vi "Setup measurement.vi"(7 "PLC (2)":dbl=2.0 format="%#_13g", 8 "error in (no error)":errorcluster, 10 "Source Limit Level (0.1)":dbl=0.1, 11 "VISA Refnum in":refnum<visa-resource-name>) -> (0 "error in (no error) 2":errorcluster, 3 "VISA resource name out":refnum<visa-resource-name>)   [LabVIEW 2021]
uses:
  <instrlib>/Keithley 2450/Keithley 2450.lvlib
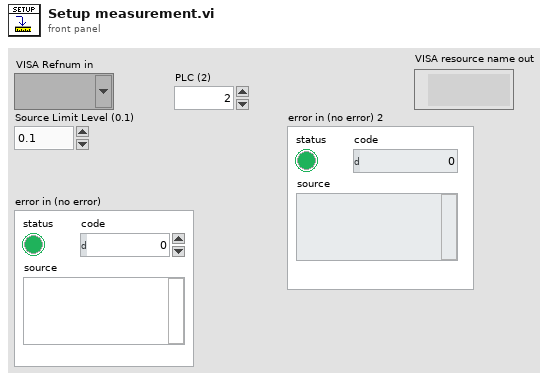
[diagram p1: front panel]
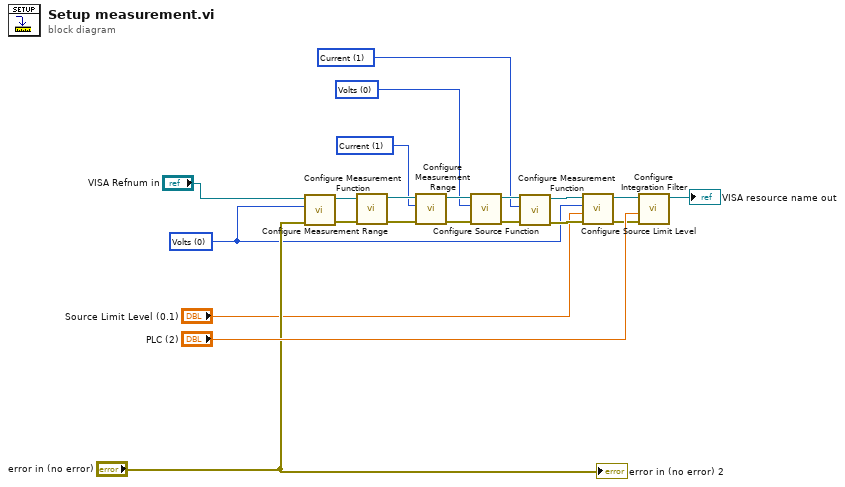
[diagram p0: block diagram]
diagram:
  w3 = u16 1 items=["Volts", "Current", "Resistance"] ("Function (0: Volts)")
  w5 = u16 0 items=["Volts", "Current"] ("Function (0: Volts)")
  w6 = u16 1 items=["Volts", "Current", "Auto Resistance", "Manual Resistance", "Digitize Voltage", "Digitize Current"] ("Function (0: Volts)")
  w4 = u16 0 items=["Volts", "Current", "Auto Resistance", "Manual Resistance", "Digitize Voltage", "Digitize Current"] ("Function (0: Volts)")
  n1 = call <instrlib>:"Configure Measurement Function.vi"("error in (no error)"="error in (no error)", "Function (0: Volts)"=w4, "VISA resource name"="VISA Refnum in") -> ("error out"=w12:errorcluster, "VISA resource name out"=w13:refnum<visa-resource-name>)  [unwired: 7 in]
  n2 = call <instrlib>:"Configure Measurement Range.vi"("error in (no error)"=w12, "VISA resource name"=w13) -> ("error out"=w10:errorcluster, "VISA resource name out"=w11:refnum<visa-resource-name>)  [unwired: 8 in]
  n3 = call <instrlib>:"Configure Measurement Range.vi"("error in (no error)"=w10, "Function (0: Volts)"=w3, "VISA resource name"=w11) -> ("error out"=w14:errorcluster, "VISA resource name out"=w15:refnum<visa-resource-name>)  [unwired: 7 in]
  n4 = call <instrlib>:"Configure Source Function.vi"("error in (no error)"=w14, "Function (0: Volts)"=w5, "VISA resource name"=w15) -> ("error out"=w19:errorcluster, "VISA resource name out"=w16:refnum<visa-resource-name>)  [unwired: 7 in]
  n5 = call <instrlib>:"Configure Measurement Function.vi"("error in (no error)"=w19, "Function (0: Volts)"=w6, "VISA resource name"=w16) -> ("error out"=w18:errorcluster, "VISA resource name out"=w17:refnum<visa-resource-name>)  [unwired: 7 in]
  n6 = call <instrlib>:"Configure Source Limit Level.vi"("error in (no error)"=w18, "Source Limit (1.0)"="Source Limit Level (0.1)", "Function (0: Volts)"=w4, "VISA resource name"=w17) -> ("error out"=w1:errorcluster, "VISA resource name out"=w7:refnum<visa-resource-name>)  [unwired: 6 in]
  n7 = call <instrlib>:"Configure Integration Filter.vi"("error in (no error)"=w1, "Measurement Speed (1 PLC)"="PLC (2)", "VISA resource name"=w7) -> ("VISA resource name out"=→"VISA resource name out":refnum<visa-resource-name>)  [unwired: 7 in, 1 out]
  "error in (no error) 2" <- "error in (no error)"
